vi "Destroy.vi"(0 "reference":refnum<class "PointNode.lvclass">, 5 "error in (no error)":errorcluster) -> (14 "reference out":refnum<class "PointNode.lvclass">, 19 "error out":errorcluster)   [LabVIEW 2016, in "PointNode.lvclass"]
doc: "Destroys a PointNode object created with a PointNode constructor VI.\n\n[GOOP 2.1]"
uses:
  <resource>/Framework/Providers/Open_GDS/UML/PointNode_class/PointNode.lvclass
  <resource>/Framework/Providers/Open_GDS/UML/AbstractNode_class/AbstractNode.lvclass
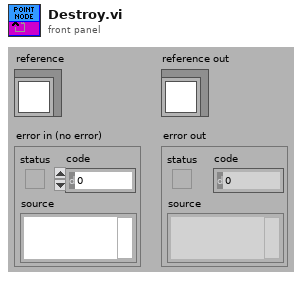
[diagram p1: front panel]
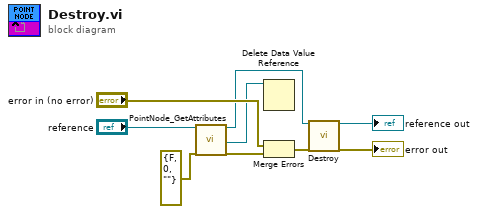
[diagram p0: block diagram]
diagram:
  n1 = call <resource>:"PointNode_GetAttributes.vi"("reference in"="reference", "error in (no error)"=errorcluster {"status"=FALSE, "code"=0, "source"=""}) -> ("reference out"=w2:refnum<class "PointNode.lvclass">, "DataRef"=w3:refnum<data-value>, "error out"=w5:errorcluster)  [unwired: 1 in, 14 out]
  n2 = Delete Data Value Reference(data value reference=w3) -> ()  [unwired: 1 in, 2 out]
  n3 = Merge Errors("error in (no error)", w5) -> (w4:errorcluster)
  n4 = call-parent "Destroy.vi"("reference"=w2, "error in (no error)"=w4) -> ("reference out"=→"reference out":refnum<class "PointNode.lvclass">, "error out"=→"error out":errorcluster)  [unwired: 16 in]
